vi "Rotation stage shgv7.vi"() -> ()   [LabVIEW 2020]
doc: "Shows how to move a motor to an absolute position."
uses:
  <vilib>/Utility/error.llb/DialogType.ctl
  <vilib>/DAQmx/read.llb/DAQmx Read (Analog 1D Wfm NChan 1Samp).vi
  <vilib>/DAQmx/read.llb/DAQmx Read (Counter 1D U32 1Chan NSamp).vi
  <vilib>/DAQmx/create/channels.llb/DAQmx Create Channel (CI-Period).vi
  <vilib>/DAQmx/create/channels.llb/DAQmx Create Channel (CO-Pulse Generation-Frequency).vi
  <vilib>/DAQmx/configure/timing.llb/DAQmx Timing (Implicit).vi
  <vilib>/DAQmx/miscellaneous.llb/DAQmx Fill In Error Info.vi
  <vilib>/DAQmx/create/channels.llb/DAQmx Create Channel (AI-Current-Basic).vi
  <vilib>/DAQmx/configure/timing.llb/DAQmx Timing (Sample Clock).vi
  <resource>/objmgr/daqmx.rc
panel:
  in  "Rotation Angle (Degrees)":dbl=100.0 min=0.0
  in  "MG17Motor":refnum<k7>(container)
  out "Actual Sample Rate":dbl=1000.0 format="%0.2f"
  out "data 2":waveform(dbl)[](graph)
  out "Consumer Iteration 3":i32=1109257
  in  "stop 4":bool
  out "Producer Iteration 3":i32=1109256
  out "error out 3":errorcluster
  out "Loop Time (ms) 3":u32=10
  in  "Duty Cycle":dbl=0.5 format="%.6f"
  out "Input.BufSize":u32=1000000 format="%.0p"
  out "data":u32[](graph)
  out "Consumer Iteration 2":i32=1109257
  in  "stop 3":bool
  in  "number of samples per channel 2":i32=5000
  out "Producer Iteration 2":i32=1109256
  out "error out 2":errorcluster
  out "Loop Time (ms) 2":u32=10
  in  "dwell time (ms)":dbl=1.0 format="%.6f"
  in  "Photon Input (PFI)":tag="/Dev1/PFI0"
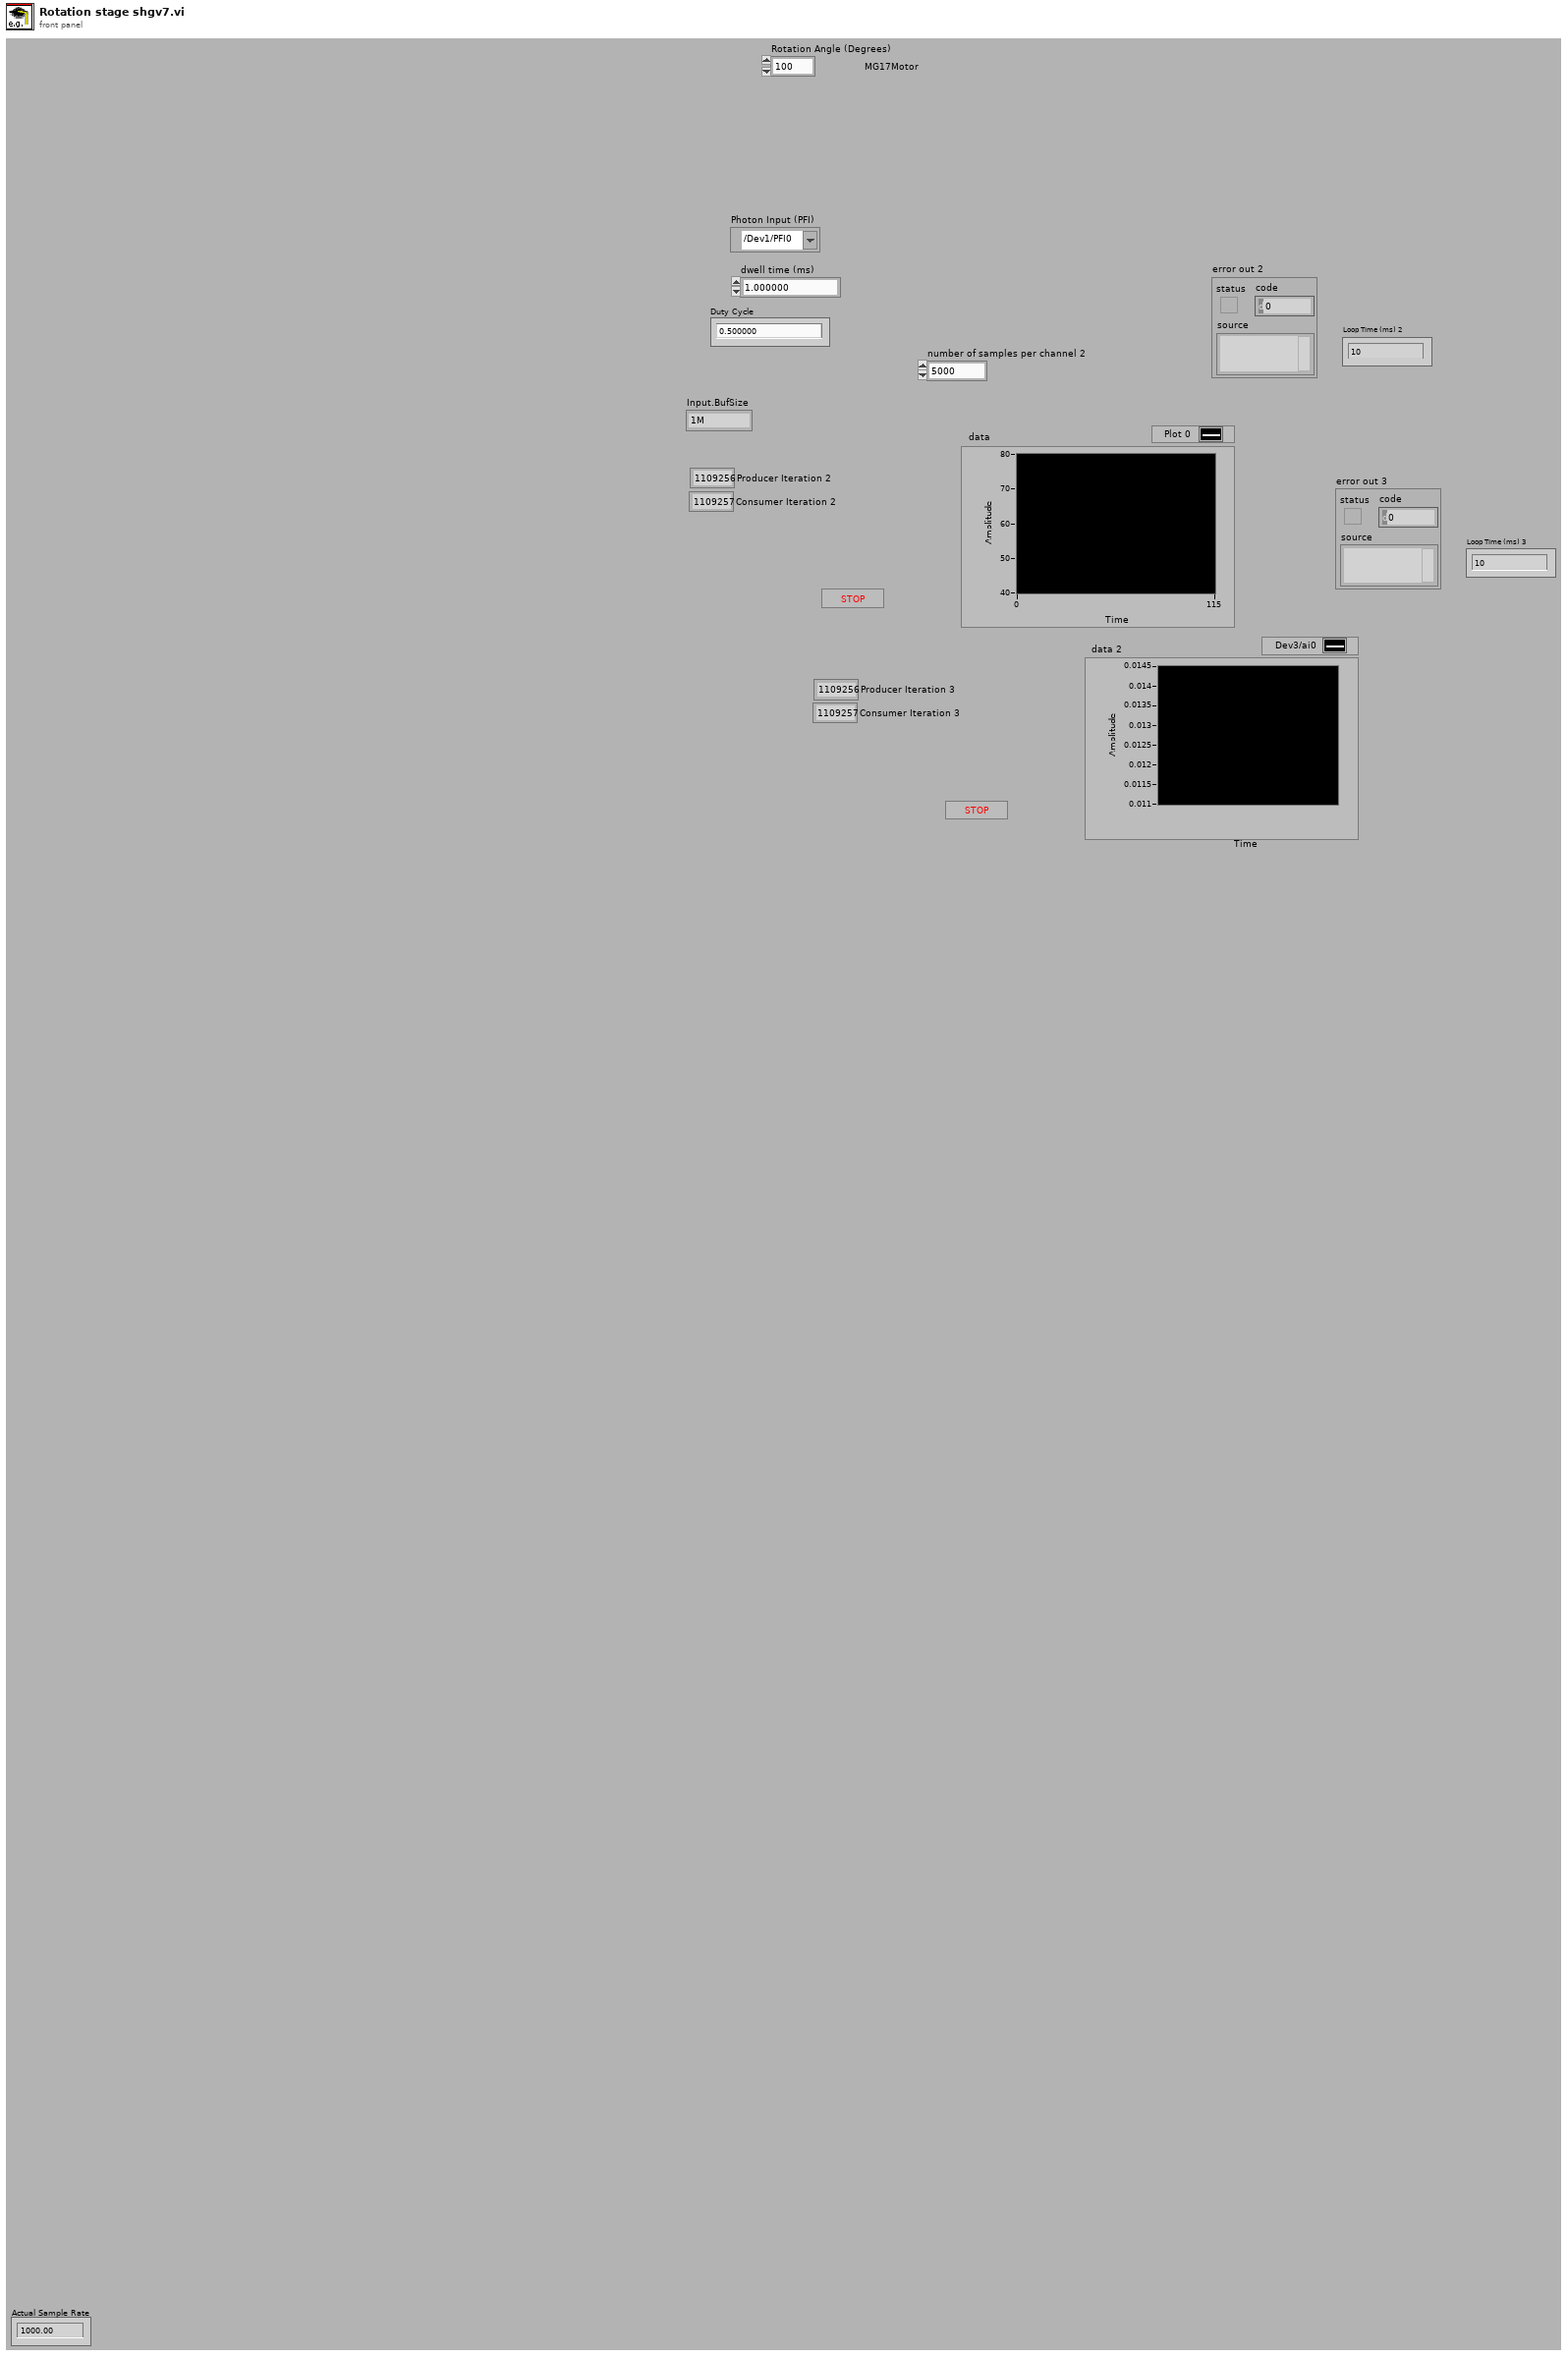
[diagram p1: front panel]
types:
  T1 = enum16{"open", "open or create", "create or replace", "create", "open (read-only)"}
  T2 = typedef "DialogType.ctl" = u16
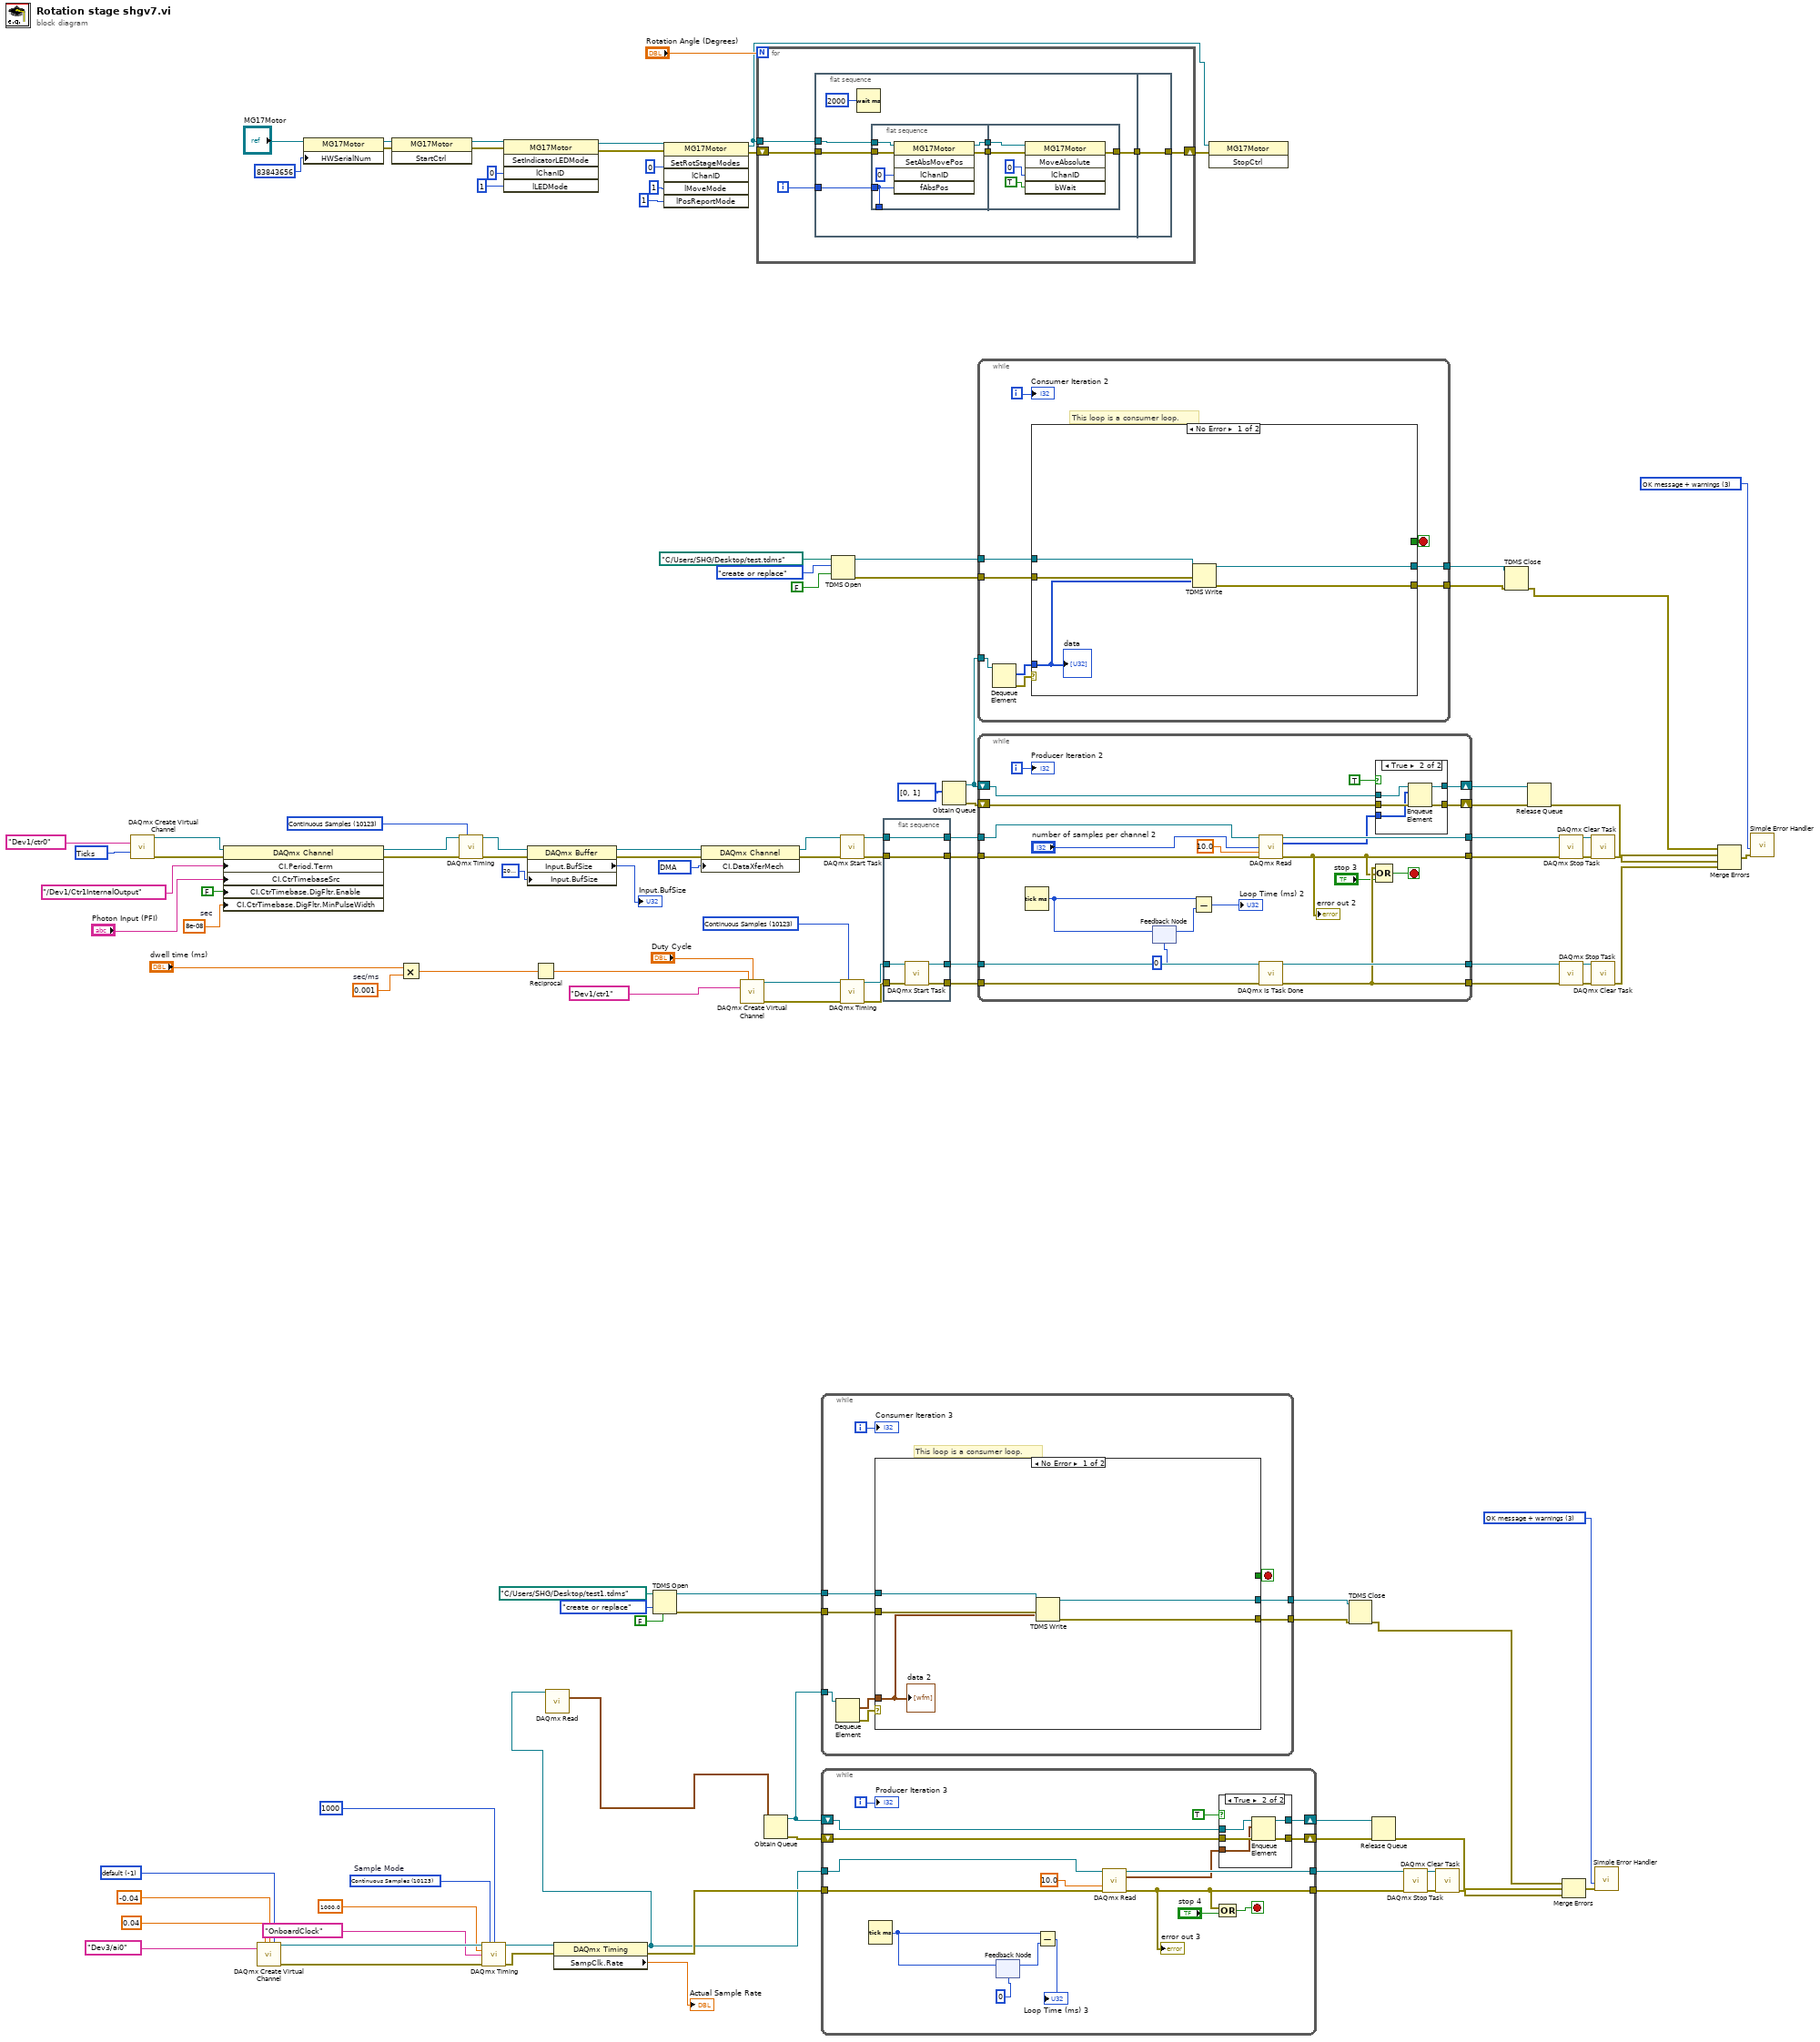
[diagram p0: block diagram]
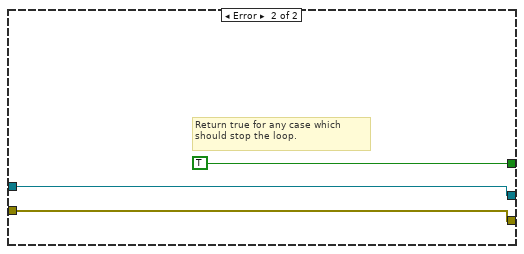
[diagram p2: hidden frame]
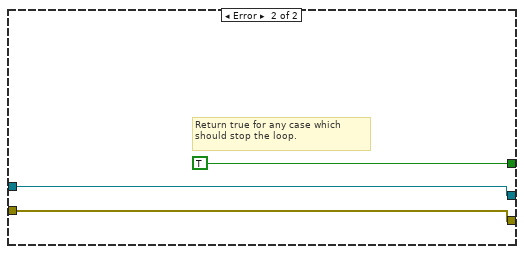
[diagram p4: hidden frame]
diagram:
  w23 = -1 items=["default"=-1, "RSE"=10083, "NRSE"=10078, "Differential"=10106, "Pseudodifferential"=12529] ("Terminal Configuration")
  w31 = 10123 items=["Finite Samples"=10178, "Continuous Samples"=10123, "Hardware Timed Single Point"=12522]  # Sample Mode
  w41 = T2 3 items=["no dialog", "OK message", "continue or stop message", "OK message + warnings", "continue/stop + warnings"] ("type of dialog (OK msg:1)")
  w62 = T2 3 items=["no dialog", "OK message", "continue or stop message", "OK message + warnings", "continue/stop + warnings"] ("type of dialog (OK msg:1)")
  w67 = 8e-08  # sec
  w78 = 10054 items=["DMA"=10054, "Interrupts"=10204, "Programmed I/O"=10264, "USB Bulk"=12590] ("CI.DataXferMech")
  w98 = 0.001  # sec/ms
  w108 = 10304 items=["Seconds"=10364, "Ticks"=10304, "From Custom Scale"=10065] ("units")
  w109 = 10123 items=["Finite Samples"=10178, "Continuous Samples"=10123, "Hardware Timed Single Point"=12522] ("sample mode")
  w110 = 10123 items=["Finite Samples"=10178, "Continuous Samples"=10123, "Hardware Timed Single Point"=12522] ("sample mode")
  n1 = call-poly <vilib>:"DAQmx Create Virtual Channel.vi"("counter"=tag "Dev1/ctr0", "units"=w108) -> ("task out"=w105:refnum<k21>, "error out"=w104:errorcluster)  [unwired: 12 in]
  n2 = property class="DAQmx Channel"(reference=w105, error in=w104, "CI.Period.Term"=tag "/Dev1/Ctr1InternalOutput", "CI.CtrTimebaseSrc"="Photon Input (PFI)", "CI.CtrTimebase.DigFltr.Enable"=FALSE, "CI.CtrTimebase.DigFltr.MinPulseWidth"=w67) -> (reference out=w103:refnum<k21>, error out=w102:errorcluster)
  n3 = call-poly <vilib>:"DAQmx Create Virtual Channel.vi"("maximum value"=0.04 ("Max Voltage"), "minimum value"=-0.04 ("Min Voltage"), "input terminal configuration"=w23, "physical channels"=tag "Dev3/ai0" ("Physical Channel")) -> ("task out"=w29:refnum<k21>, "error out"=w30:errorcluster)  [unwired: 10 in]
  n4 = property class="MG17Motor"(reference="MG17Motor", "HWSerialNum"=83843656) -> (reference out=w15:refnum<k7>, error out=w14:errorcluster)  [unwired: 1 in]
  n5 = invoke class="MG17Motor" method="StartCtrl"(reference=w15, error in=w14) -> (reference out=w6:refnum<k7>, error out=w4:errorcluster)  [unwired: 1 in, 1 out]
  n6 = Multiply(x="dwell time (ms)", y=w98) -> (x*y=w97:dbl)
  n7 = call-poly <vilib>:"DAQmx Timing.vi"("task/channels in"=w103, "sample mode"=w109, "error in"=w102) -> ("task out"=w73:refnum<k21>, "error out"=w72:errorcluster)  [unwired: 11 in]
  n8 = call-poly <vilib>:"DAQmx Timing.vi"("task/channels in"=w29, "sample mode"=w31, "samples per channel"=1000 ("Number of Samples"), "rate"=1000.0 ("Sample Rate"), "source"=tag "OnboardClock" ("Sample Clock Source"), "error in"=w30) -> ("task out"=w33:refnum<k21>, "error out"=w32:errorcluster)  [unwired: 8 in]
  n9 = invoke class="MG17Motor" method="SetIndicatorLEDMode"(reference=w6, error in=w4, "lChanID"=0, "lLEDMode"=1) -> (reference out=w5:refnum<k7>, error out=w3:errorcluster)  [unwired: 1 in, 3 out]
  n10 = property class="DAQmx Buffer"(reference=w73, error in=w72, "Input.BufSize"=u32 2000000 ("samples per channel")) -> (reference out=w77:refnum<k21>, error out=w75:errorcluster, "Input.BufSize"=→"Input.BufSize":u32)
  n11 = Reciprocal(x=w97) -> (1/x=w96:dbl)
  n12 = property class="DAQmx Timing"(reference=w33, error in=w32) -> (reference out=w18:refnum<k21>, error out=w27:errorcluster, "SampClk.Rate"=→"Actual Sample Rate":dbl)
  n13 = call-poly <vilib>:"DAQmx Read.vi"("task/channels in"=w18) -> ("data"=w19:waveform(dbl)[])  [unwired: 12 in, 2 out]
  n14 = TDMS Open(6:FALSE ("disable buffering? (T)"), 10:T1."create or replace" ("operation (0:open)"), 11:path "C:/Users/SHG/Desktop/test1.tdms" ("file path")) -> (0:w43:errorcluster, 3:w45:refnum<k34>)  [unwired: 4 in]
  n15 = invoke class="MG17Motor" method="SetRotStageModes"(reference=w5, error in=w3, "lChanID"=0, "lMoveMode"=1, "lPosReportMode"=1) -> (reference out=w9:refnum<k7>, error out=w10:errorcluster)  [unwired: 1 in, 4 out]
  n16 = property class="DAQmx Channel"(reference=w77, error in=w75, "CI.DataXferMech"=w78) -> (reference out=w71:refnum<k21>, error out=w70:errorcluster)
  n17 = call-poly <vilib>:"DAQmx Create Virtual Channel.vi"("frequency"=w96, "duty cycle"="Duty Cycle", "counter"=tag "Dev1/ctr1") -> ("task out"=w115:refnum<k21>, "error out"=w116:errorcluster)  [unwired: 11 in]
  n18 = for {
    N: "Rotation Angle (Degrees)" -> [_]
    tunnel: w9 -> [w121]
    shift-right: [w119] -> w17
    shift-left: w10 -> [w120]
    i -> [w117]
    n19 = flat-sequence {
      tunnel: w121 -> [w126]
      tunnel: w120 -> [w124]
      tunnel: [w123] -> w118
      tunnel: w117 -> [w125]
      tunnel: [w140] -> w119
      tunnel: w118 -> [w140]
      frame #0 {
        n20 = Wait (ms)(milliseconds to wait=u32 2000) -> ()  [unwired: 1 out]
        n21 = flat-sequence {
          tunnel: [w129] -> _
          tunnel: w124 -> [w133]
          tunnel: w126 -> [w132]
          tunnel: [w131] -> w128
          tunnel: [w130] -> w127
          tunnel: w125 -> [w129]
          tunnel: w128 -> [w137]
          tunnel: w127 -> [w136]
          tunnel: [w135] -> w123
          frame #0 {
            n22 = invoke class="MG17Motor" method="SetAbsMovePos"(reference=w132, error in=w133, "lChanID"=0, "fAbsPos"=w129) -> (reference out=w130:refnum<k7>, error out=w131:errorcluster)  [unwired: 1 in, 3 out]
          }
          frame #1 {
            n23 = invoke class="MG17Motor" method="MoveAbsolute"(reference=w136, error in=w137, "lChanID"=0, "bWait"=TRUE) -> (error out=w135:errorcluster)  [unwired: 1 in, 4 out]
          }
        }
      }
      frame #1 {
      }
    }
  }
  n24 = Obtain Queue(element data type=w19) -> (queue out=w53:refnum<queue>, error out=w52:errorcluster)  [unwired: 4 in, 1 out]
  n25 = while {
    tunnel: w53 -> [w149]
    tunnel: w45 -> [w144]
    tunnel: [w143] -> w44
    tunnel: w43 -> [w142]
    tunnel: [w141] -> w42
    i -> [w145]
    stop <- w146 stop-if-true
    # "This loop is a consumer loop."
    n26 = Dequeue Element(queue=w149) -> (element=w147:waveform(dbl)[], error out=w148:errorcluster)  [unwired: 2 in, 2 out]
    n27 = case shown="No Error" w148 {
      tunnel: w147 -> [w150 _]
      tunnel: [_ TRUE] -> w146
      tunnel: w144 -> [w154 w156]
      tunnel: [w153 w156] -> w143
      tunnel: w142 -> [w152 w155]
      tunnel: [w151 w155] -> w141
      frame No Error {
        n28 = TDMS Write(0:w154, 9:w150, 11:w152) -> (4:w153:refnum<k34>, 15:w151:errorcluster)  [unwired: 3 in, 2 out]
        "data 2" <- w150
      }
      frame Error {
        # "Return true for any case which should stop the loop."
      }
    }
    "Consumer Iteration 3" <- w145
  }
  n29 = while {
    shift-right: [w165] -> w50
    shift-left: w52 -> [w173]
    shift-right: [w174] -> w51
    shift-left: w53 -> [w175]
    tunnel: [w171] -> w47
    tunnel: [w164] -> w46
    tunnel: w27 -> [w170]
    tunnel: w18 -> [w169]
    i -> [w166]
    stop <- w162 stop-if-true
    n30 = Tick Count (ms)() -> (millisecond timer value=w161:u32)
    n31 = feedback #1(u32 0 ("millisecond timer value")) -> (w160:u32)
    n32 = feedback-in #1(w161) -> ()
    n33 = Subtract(x=w161, y=w160) -> (x-y=→"Loop Time (ms) 3":u32)
    n34 = call-poly <vilib>:"DAQmx Read.vi"("task/channels in"=w169, "timeout"=10.0, "error in"=w170) -> ("task out"=w171:refnum<k21>, "data"=w168:waveform(dbl)[], "error out"=w164:errorcluster)  [unwired: 10 in]
    "error out 3" <- w164
    n35 = case shown="True" TRUE ("Case Constant\n(See Context Help)") {
      tunnel: w175 -> [w177 w182]
      tunnel: [w177 w181] -> w174
      tunnel: w173 -> [w176 w180]
      tunnel: [w176 w179] -> w165
      tunnel: w168 -> [_ w178]
      frame False {
      }
      frame True {
        n36 = Enqueue Element(queue=w182, element=w178, error in (no error)=w180) -> (queue out=w181:refnum<queue>, error out=w179:errorcluster)  [unwired: 1 in, 1 out]
      }
    }
    n37 = Compound Arithmetic op=OR(w164, "stop 4") -> (w162:bool)
    "Producer Iteration 3" <- w166
  }
  n38 = TDMS Open(6:FALSE ("disable buffering? (T)"), 10:T1."create or replace" ("operation (0:open)"), 11:path "C:/Users/SHG/Desktop/test.tdms" ("file path")) -> (0:w64:errorcluster, 3:w66:refnum<k34>)  [unwired: 4 in]
  n39 = call <vilib>:"DAQmx Start Task.vi"("task/channels in"=w71, "error in"=w70) -> ("task out"=w95:refnum<k21>, "error out"=w94:errorcluster)  [unwired: 12 in]
  n40 = call-poly <vilib>:"DAQmx Timing.vi"("task/channels in"=w115, "sample mode"=w110, "error in"=w116) -> ("task out"=w114:refnum<k21>, "error out"=w113:errorcluster)  [unwired: 11 in]
  n41 = flat-sequence {
    tunnel: w114 -> [w188]
    tunnel: w113 -> [w187]
    tunnel: [w186] -> w81
    tunnel: [w185] -> w82
    tunnel: w95 -> [w183]
    tunnel: w94 -> [w184]
    tunnel: [w184] -> w84
    tunnel: [w183] -> w83
    frame #0 {
      n42 = call <vilib>:"DAQmx Start Task.vi"("task/channels in"=w188, "error in"=w187) -> ("task out"=w185:refnum<k21>, "error out"=w186:errorcluster)  [unwired: 12 in]
    }
  }
  n43 = Obtain Queue(element data type=u32[] [0, 1] ("data")) -> (queue out=w93:refnum<queue>, error out=w92:errorcluster)  [unwired: 4 in, 1 out]
  n44 = while {
    tunnel: w93 -> [w197]
    tunnel: w66 -> [w192]
    tunnel: [w191] -> w65
    tunnel: w64 -> [w190]
    tunnel: [w189] -> w63
    i -> [w193]
    stop <- w194 stop-if-true
    # "This loop is a consumer loop."
    n45 = Dequeue Element(queue=w197) -> (element=w195:u32[], error out=w196:errorcluster)  [unwired: 2 in, 2 out]
    n46 = case shown="No Error" w196 {
      tunnel: w195 -> [w198 _]
      tunnel: [_ TRUE] -> w194
      tunnel: w192 -> [w202 w204]
      tunnel: [w201 w204] -> w191
      tunnel: w190 -> [w200 w203]
      tunnel: [w199 w203] -> w189
      frame No Error {
        n47 = TDMS Write(0:w202, 9:w198, 11:w200) -> (4:w201:refnum<k34>, 15:w199:errorcluster)  [unwired: 3 in, 2 out]
        "data" <- w198
      }
      frame Error {
        # "Return true for any case which should stop the loop."
      }
    }
    "Consumer Iteration 2" <- w193
  }
  n48 = while {
    shift-right: [w217] -> w90
    shift-left: w92 -> [w226]
    shift-right: [w227] -> w91
    shift-left: w93 -> [w228]
    tunnel: [w224] -> w87
    tunnel: [w212] -> w86
    tunnel: w84 -> [w223]
    tunnel: w83 -> [w222]
    tunnel: w82 -> [w216]
    tunnel: w81 -> [w215]
    tunnel: [w214] -> w80
    tunnel: [w213] -> w79
    i -> [w218]
    stop <- w210 stop-if-true
    n49 = Tick Count (ms)() -> (millisecond timer value=w209:u32)
    n50 = feedback #2(u32 0 ("millisecond timer value")) -> (w208:u32)
    n51 = feedback-in #2(w209) -> ()
    n52 = Subtract(x=w209, y=w208) -> (x-y=→"Loop Time (ms) 2":u32)
    n53 = call-poly <vilib>:"DAQmx Read.vi"("task/channels in"=w222, "number of samples per channel"="number of samples per channel 2", "timeout"=10.0, "error in"=w223) -> ("task out"=w224:refnum<k21>, "data"=w221:u32[], "error out"=w212:errorcluster)  [unwired: 9 in]
    "error out 2" <- w212
    n54 = call <vilib>:"DAQmx Is Task Done.vi"("task/channels in"=w216, "error in"=w215) -> ("task out"=w214:refnum<k21>, "error out"=w213:errorcluster)  [unwired: 11 in, 1 out]
    n55 = case shown="True" TRUE ("Case Constant\n(See Context Help)") {
      tunnel: w228 -> [w230 w235]
      tunnel: [w230 w234] -> w227
      tunnel: w226 -> [w229 w233]
      tunnel: [w229 w232] -> w217
      tunnel: w221 -> [_ w231]
      frame False {
      }
      frame True {
        n56 = Enqueue Element(queue=w235, element=w231, error in (no error)=w233) -> (queue out=w234:refnum<queue>, error out=w232:errorcluster)  [unwired: 1 in, 1 out]
      }
    }
    n57 = Compound Arithmetic op=OR(w213, w212, "stop 3") -> (w210:bool)
    "Producer Iteration 2" <- w218
  }
  n58 = invoke class="MG17Motor" method="StopCtrl"(reference=w9, error in=w17) -> ()  [unwired: 1 in, 3 out]
  n59 = TDMS Close(8:w42, 11:w44) -> (0:w37:errorcluster)  [unwired: 1 out]
  n60 = Release Queue(queue=w51, error in (no error)=w50) -> (error out=w36:errorcluster)  [unwired: 1 in, 2 out]
  n61 = call <vilib>:"DAQmx Stop Task.vi"("task/channels in"=w47, "error in"=w46) -> ("task out"=w48:refnum<k21>, "error out"=w49:errorcluster)  [unwired: 12 in]
  n62 = call <vilib>:"DAQmx Clear Task.vi"("task in"=w48, "error in"=w49) -> ("error out"=w35:errorcluster)  [unwired: 13 in]
  n63 = TDMS Close(8:w63, 11:w65) -> (0:w58:errorcluster)  [unwired: 1 out]
  n64 = Release Queue(queue=w91, error in (no error)=w90) -> (error out=w57:errorcluster)  [unwired: 1 in, 2 out]
  n65 = call <vilib>:"DAQmx Stop Task.vi"("task/channels in"=w87, "error in"=w86) -> ("task out"=w88:refnum<k21>, "error out"=w89:errorcluster)  [unwired: 12 in]
  n66 = call <vilib>:"DAQmx Stop Task.vi"("task/channels in"=w80, "error in"=w79) -> ("task out"=w112:refnum<k21>, "error out"=w111:errorcluster)  [unwired: 12 in]
  n67 = Merge Errors(w37, w36, w35) -> (w40:errorcluster)
  n68 = call <vilib>:"DAQmx Clear Task.vi"("task in"=w88, "error in"=w89) -> ("error out"=w56:errorcluster)  [unwired: 13 in]
  n69 = call <vilib>:"DAQmx Clear Task.vi"("task in"=w112, "error in"=w111) -> ("error out"=w55:errorcluster)  [unwired: 13 in]
  n70 = call <vilib>:"Simple Error Handler.vi"("type of dialog (OK msg:1)"=w41, "error in (no error)"=w40) -> ()  [unwired: 3 in, 5 out]
  n71 = Merge Errors(w58, w57, w56, w55) -> (w61:errorcluster)
  n72 = call <vilib>:"Simple Error Handler.vi"("type of dialog (OK msg:1)"=w62, "error in (no error)"=w61) -> ()  [unwired: 3 in, 5 out]
